vi "Write U8 Array.vi"(8 "error in":errorcluster, 9 "Cluster BLOB in":u8[](array[numeric]), 10 "register name":string, 11 "session in":u32) -> (0 "error out":errorcluster, 3 "session out":u32)   [LabVIEW 2018, in "Scalar IO Operations.lvlib"]
uses:
  Scalar IO Operations.lvlib
  NiFpga.dll
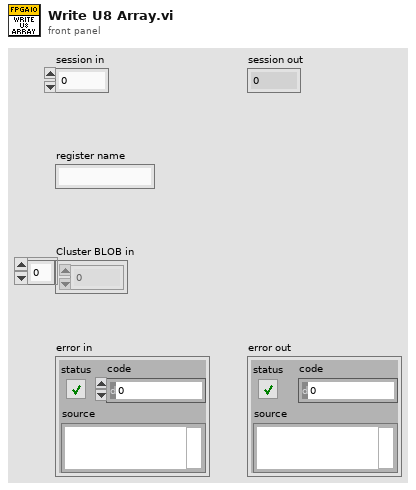
[diagram p1: front panel]
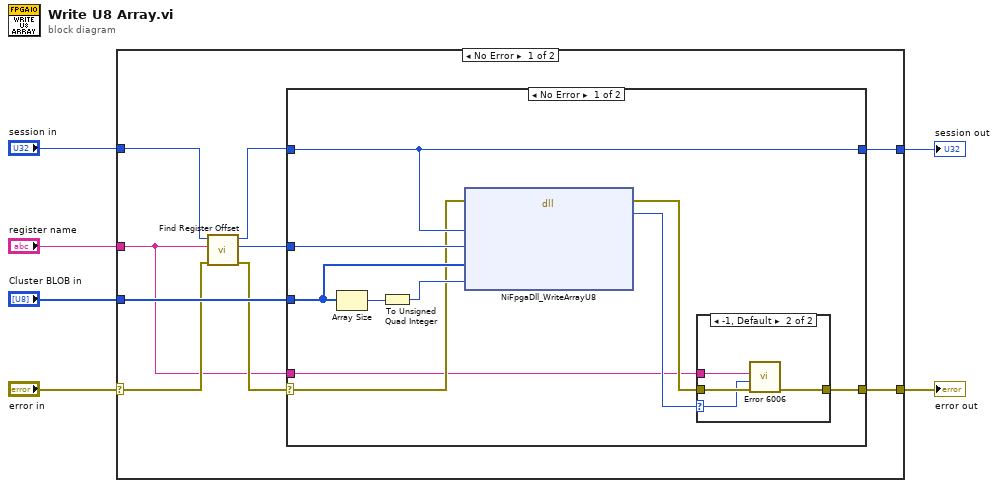
[diagram p0: block diagram]
diagram:
  n1 = case shown="No Error" "error in" {
    selector: "error in" -> [w11 w33]
    tunnel: "session in" -> [w12 w34]
    tunnel: [w15 w33] -> w5
    tunnel: [w14 w34] -> w4
    tunnel: "Cluster BLOB in" -> [w13 _]
    tunnel: "register name" -> [w7 _]
    frame No Error {
      n2 = call "Find Register Offset.vi"("error in (no error)"=w11, "register name"=w7, "session in"=w12) -> ("error out"=w10:errorcluster, "resource offset"=w9:u32, "session out"=w8:u32)  [unwired: 6 in]
      n3 = case shown="No Error" w10 {
        selector: w10 -> [w20 w32]
        tunnel: w8 -> [w25 w31]
        tunnel: [w19 w32] -> w15
        tunnel: w9 -> [w24 _]
        tunnel: [w25 w31] -> w14
        tunnel: w13 -> [w23 _]
        tunnel: w7 -> [w16 _]
        frame No Error {
          n4 = Array Size(array=w23) -> (size(s)=w22:i32)
          n5 = To Unsigned Quad Integer(1:w22) -> (0:w21:u64)
          n6 = dll-call lib="NiFpga.*" fn="NiFpgaDll_WriteArrayU8"(error in=w20, "session"=w25, "offset"=w24, "data"=w23, "count"=w21) -> (error out=w18:errorcluster, "status"=w17:i32)  [unwired: 6 in, 1 out]
          n7 = case shown="-1, Default" w17 {
            selector: w17 -> [_ w28]
            tunnel: w18 -> [w26 w29]
            tunnel: [w26 w30] -> w19
            tunnel: w16 -> [_ w27]
            frame 0 {
            }
            frame -1, Default {
              n8 = call "Error 6006.vi"("error in (no error)"=w29, "rio status code"=w28, "register name"=w27) -> ("error out"=w30:errorcluster)  [unwired: 8 in]
            }
          }
        }
        frame Error {
        }
      }
    }
    frame Error {
    }
  }
  "error out" <- w5
  "session out" <- w4
